vi "To 2D Float Tree Data.vi"(10 "2D Flt":dbl[][](array[numeric])) -> (3 "2D Flt Tree Data":refnum<class "2D Flt.lvclass">)   [LabVIEW 2017, in "Tree API.lvlib" / "2D Flt.lvclass"]
doc: "Convert a 1D Float value to Tree Data type."
uses:
  2D Flt.lvclass
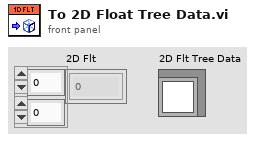
[diagram p1: front panel]
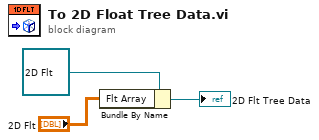
[diagram p0: block diagram]
diagram:
  n1 = Bundle By Name(cluster=refnum<class "2D Flt.lvclass"> refnum ("Tree API.lvlib:2D Flt.lvclass"), "Flt Array"="2D Flt") -> (→"2D Flt Tree Data":refnum<class "2D Flt.lvclass">)
